vi "_Read XML Table.vi"(4 "error in":errorcluster, 7 "XML String":string) -> (0 "error out":errorcluster, 1 "Table Type":i32, 2 "Table (2D-DBL)":dbl[][](array[numeric]), 3 "Remaining String":string)   [LabVIEW 2015]
uses:
  Type/_XML Type.ctl
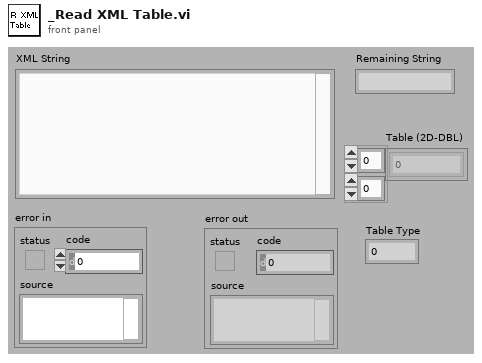
[diagram p1: front panel]
types:
  T1 = typedef "_XML Type.ctl" = enum16{"Configuration", "ConTable", "Method", "Experiment", "Mass Range", "Table", "LensTable", "ParamTable", "TuneParam", "MetParam", "MassRange", "LCMethod", "LCMethodFile", "RackType", "Vial", "PlatePos", "InjVol"}
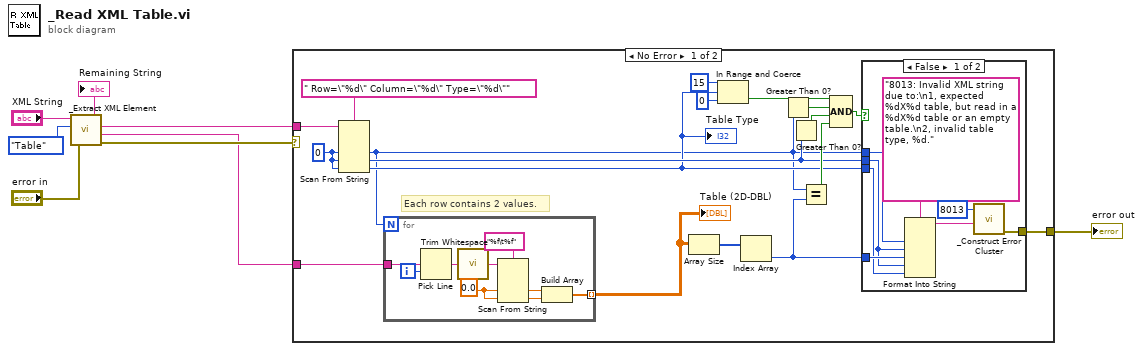
[diagram p0: block diagram]
diagram:
  n1 = call "_Extract XML Element.vi"("error in"="error in", "XML Type"=_XML_Type."Table", "XML String"="XML String") -> ("error out"=w3:errorcluster, "Element"=w1:string, "Attributes"=w2:string, "Remaining String"=→"Remaining String":string)  [unwired: 1 out]
  n2 = case shown="No Error" w3 {
    selector: w3 -> [_ w44]
    tunnel: w2 -> [w21 _]
    tunnel: [w26 w44] -> w8
    tunnel: w1 -> [w10 _]
    frame No Error {
      w16 = 0 ("default value 1")
      # "Each row contains 2 values."
      n3 = Scan From String(format string=" Row=\"%d\" Column=\"%d\" Type=\"%d\"", input string=w21, default 1=w16, default 2=w16, default 3=w16) -> (output 1=w11:i32, output 2=w19:i32, output 3=w12:i32)  [unwired: 2 in, 3 out]
      "Table Type" <- w12
      n4 = for {
        N: w11 -> [_]
        tunnel: w10 -> [w33]
        tunnel: [w30] -> w9 mode=indexing
        i -> [w32]
        w29 = 0.0 ("Ch#")
        n5 = Pick Line(multi-line string=w33, line index=w32) -> (output string=w34:string)  [unwired: 1 out]
        n6 = call <vilib>:"Trim Whitespace.vi"("string"=w34) -> ("trimmed string"=w31:string)  [unwired: 1 in]
        n7 = Scan From String(format string="%f\t%f", input string=w31, default 1=w29, default 2=w29) -> (output 1=w28:dbl, output 2=w27:dbl)  [unwired: 2 in, 3 out]
        n8 = Build Array(w28, w27) -> (w30:dbl[])
      }
      "Table (2D-DBL)" <- w9
      n9 = Array Size(array=w9) -> (size(s)=w25:i32[])
      n10 = In Range and Coerce(upper limit=15, x=w12, lower limit=0) -> (In Range?=w13:bool)  [unwired: 1 out]
      n11 = Index Array(array=w25) -> (element=w22:i32)  [unwired: 1 in]
      n12 = Greater Than 0?(x=w11) -> (x > 0?=w17:bool)
      n13 = Greater Than 0?(x=w19) -> (x > 0?=w18:bool)
      n14 = Equal?(x=w11, y=w22) -> (x = y?=w24:bool)
      n15 = Compound Arithmetic op=AND(w13, w17, w18, w24) -> (w23:bool)
      n16 = case shown="False" w23 {
        tunnel: w19 -> [w37 _]
        tunnel: w11 -> [w42 _]
        tunnel: [w43 _] -> w26
        tunnel: w22 -> [w39 _]
        tunnel: w12 -> [w38 _]
        frame False {
          n17 = Format Into String(format string="8013: Invalid XML string due to:\n1, expected %dX%d table, but read in a %dX%d table or an empty table.\n2, invalid table type, %d.", w42, w37, w39, w37, w38) -> (resulting string=w40:string)  [unwired: 2 in, 1 out]
          n18 = call "_Construct Error Cluster.vi"("reason"=w40, "errorCode"=8013) -> ("error out"=w43:errorcluster)  [unwired: 2 in, 3 out]
        }
        frame True {
        }
      }
    }
    frame Error {
    }
  }
  "error out" <- w8
